vi "SEARCH(SubVI).vi"(0 "Image In":T2, 1 "search control In":T3={"Search Strategy"=0, "Color Sensitivity"=0, "Match Feature Mode"=0, "Minimum Score"=700.0, "Nb of Matches"=1, "Subpixel Accuracy"=FALSE, "Minimum Contrast"=10, "Match Mode"=0, "Color Score Weight"=500.0, "Rotation Angle Ranges (degrees)"=[]} {"Rotation Angle Ranges (degrees)"."?" format="%.2f"; "Rotation Angle Ranges (degrees)"."?" format="%.2f"; "Color Score Weight" min=0 max=1000 format="%.2f"; "Match Mode" items=["Shift Invariant", "Rotation Invariant"]; "Match Feature Mode" items=["Color and Shape", "Color", "Shape"]; "Color Sensitivity" items=["Low Sensitivity", "Medium Sensitivity", "High Sensitivity"]; "Search Strategy" items=["Conservative", "Balance", "Aggressive", "Very Aggressive"]}, 2 "Optional Rectangle":i32[](array[numeric]), 5 "Image Temaplate In":T2, 9 "Activar Search (T)":bool=TRUE, 11 "error in":errorcluster) -> (4 "Matches Out":T1(array[cluster]) {"Bounding Box"."y" format="%.2f"; "Bounding Box"."x" format="%.2f"; "Position"."y" format="%.2f"; "Position"."x" format="%.2f"; "Score" format="%.2f"; "Scale" format="%.2f"; "Angle" format="%.2f"}, 6 "Number of Matches Out":i32, 10 "First Call?: T/F":bool, 15 "error out":errorcluster)   [LabVIEW 2011]
doc: "Hace la busqueda (search) de una imagen template (necesaria que estuviera creada antes)."
uses:
  IMAQ Image.ctl
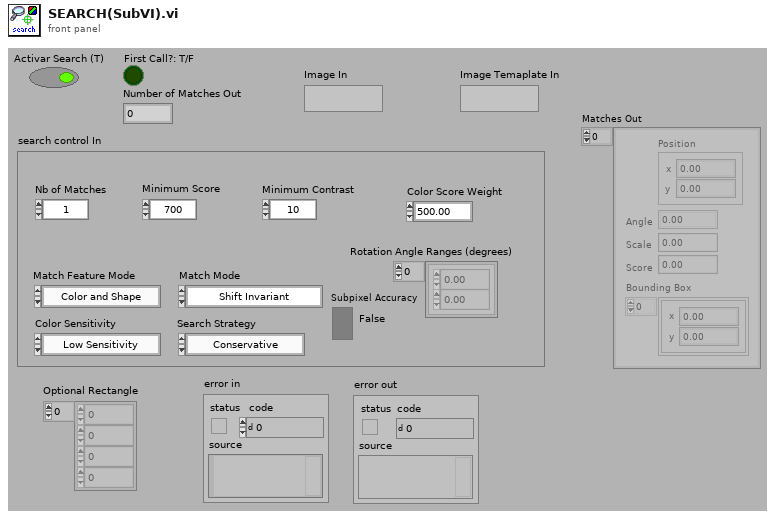
[diagram p1: front panel]
types:
  T1 = cluster{"Position":cluster{"x":sgl, "y":sgl}, "Angle":sgl, "Scale":sgl, "Score":sgl, "Bounding Box":cluster{"x":sgl, "y":sgl}[]}[]
  T2 = typedef "IMAQ Image.ctl" = cluster{string, u32}
  T3 = cluster{"Search Strategy":u32, "Color Sensitivity":u32, "Match Feature Mode":u32, "Minimum Score":sgl, "Nb of Matches":i32, "Subpixel Accuracy":bool, "Minimum Contrast":i32, "Match Mode":u16, "Color Score Weight":sgl, "Rotation Angle Ranges (degrees)":cluster{sgl, sgl}[]}
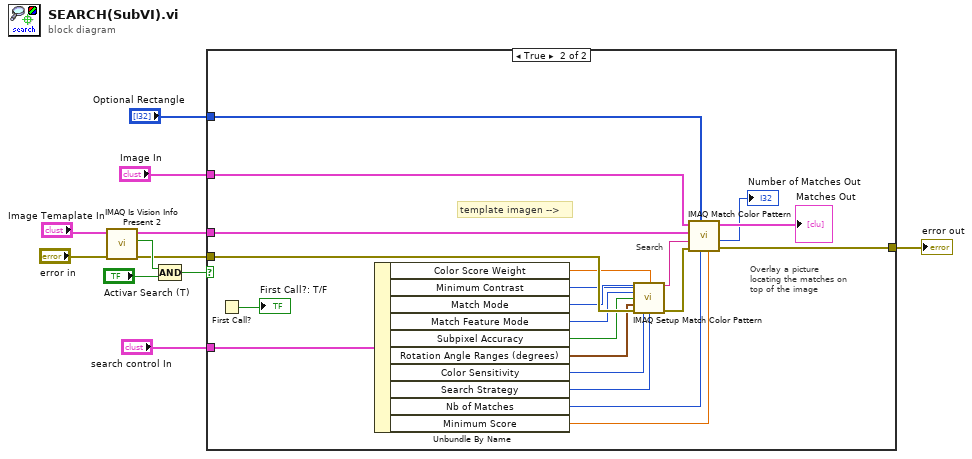
[diagram p0: block diagram]
diagram:
  n1 = call "IMAQ Is Vision Info Present 2"("error in (no error)"="error in", "Image"="Image Temaplate In") -> ("error out"=w3:errorcluster, "Present?"=w5:bool, "Image (duplicate)"=w6:T2)  [unwired: 1 in, 6 out]
  n2 = Compound Arithmetic op=AND(w5, "Activar Search (T)") -> (w8:bool)
  n3 = case shown="True" w8 {
    tunnel: "Image In" -> [_ w25]
    tunnel: w6 -> [_ w31]
    tunnel: "search control In" -> [_ w30]
    tunnel: [w12 w28] -> w9
    tunnel: w3 -> [w12 w20]
    tunnel: "Optional Rectangle" -> [_ w13]
    frame False {
    }
    frame True {
      # "template imagen -->"
      # "Overlay a picture locating the matches on top of the image"
      # "Search"
      n4 = First Call?() -> (First Call?: T/F=→"First Call?: T/F":bool)
      n5 = Unbundle By Name(w30) -> ("Color Score Weight"=w14:sgl, "Minimum Contrast"=w15:i32, "Match Mode"=w16:u16, "Match Feature Mode"=w17:u32, "Subpixel Accuracy"=w18:bool, "Rotation Angle Ranges (degrees)"=w19:cluster{sgl, sgl}[], "Color Sensitivity"=w21:u32, "Search Strategy"=w22:u32, "Nb of Matches"=w24:i32, "Minimum Score"=w23:sgl)
      n6 = call "IMAQ Setup Match Color Pattern"("Match Mode"=w16, "Minimum Contrast"=w15, "Color Score Weight"=w14, "Match Feature Mode"=w17, "Subpixel Accuracy"=w18, "Rotation Angle Ranges (degrees)"=w19, "error in (no error)"=w20, "Color Sensitivity"=w21, "Search Strategy"=w22) -> ("Match Color Pattern Setup Data"=w33:string, "error out"=w29:errorcluster)  [unwired: 5 out]
      n7 = call "IMAQ Match Color Pattern"("Minimum Match Score"=w23, "Number of Matches Requested"=w24, "Optional Rectangle"=w13, "error in (no error)"=w29, "Match Color Pattern Setup Data"=w33, "Template Image"=w31, "Image"=w25) -> ("error out"=w28:errorcluster, "Number of Matches"=→"Number of Matches Out":i32, "Matches"=→"Matches Out":T1)  [unwired: 2 out]
    }
  }
  "error out" <- w9
